vi "Read GA Options.vi"(8 "error in (no error)":errorcluster, 11 "IPopulation in":refnum<class "IPopulation.lvclass">) -> (0 "error out":errorcluster, 2 "GA Options":T1, 3 "IPopulation out":refnum<class "IPopulation.lvclass">)   [LabVIEW 2016, in "IPopulation.lvclass"]
uses:
  IPopulation.lvclass
  IPopulation.lvclass/IPopulation.ctl
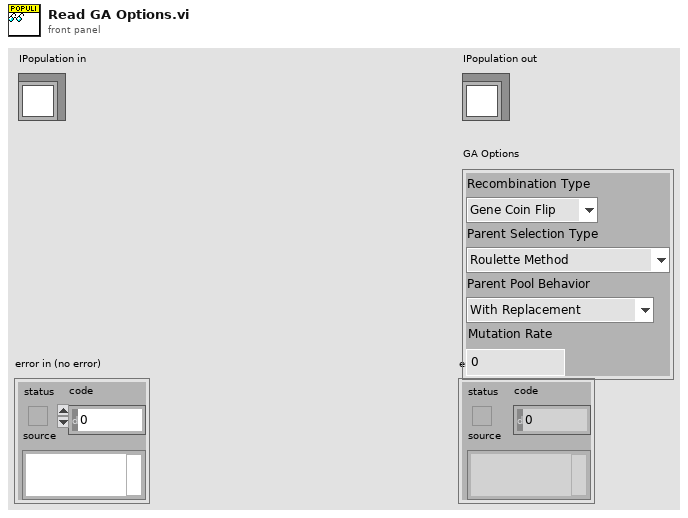
[diagram p1: front panel]
types:
  T1 = cluster{"Recombination Type":enum16{"Gene Coin Flip", "Pivot Crossover"}, "Parent Selection Type":enum16{"Roulette Method", "Rank Selection"}, "Parent Pool Behavior":enum16{"With Replacement", "Without Replacement"}, "Mutation Rate":dbl}
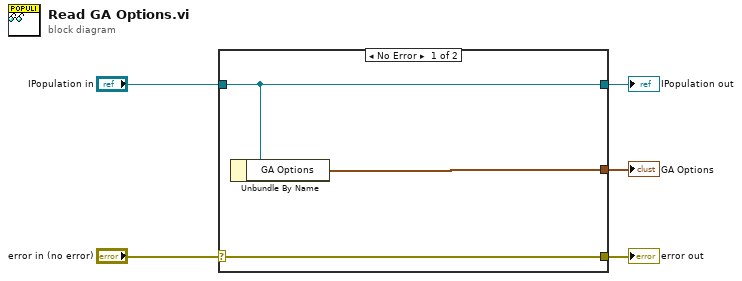
[diagram p0: block diagram]
diagram:
  n1 = case shown="No Error" "error in (no error)" {
    selector: "error in (no error)" -> [w8 w9]
    tunnel: [w8 w9] -> w4
    tunnel: [w7 w10] -> w2
    tunnel: "IPopulation in" -> [w7 w10]
    tunnel: [w6 _] -> w1
    frame No Error {
      n2 = Unbundle By Name(w7) -> ("GA Options"=w6:T1)
    }
    frame Error {
    }
  }
  "error out" <- w4
  "IPopulation out" <- w2
  "GA Options" <- w1
